vi "PCSLauncher.get Supers and Start-GOGs.vi"(0 "i ref in":refnum<vi>, 5 "error in (no error)":errorcluster) -> (14 "i ref out":refnum<vi>, 16 "Super Instances":string[](array[string]), 17 "Start-GOG Instances":string[](array[string]), 18 "System Names":string[](array[string]), 19 "error out":errorcluster)   [LabVIEW 2014, in "PCSLauncher.lvlib"]
uses:
  PCSLauncher.lvlib
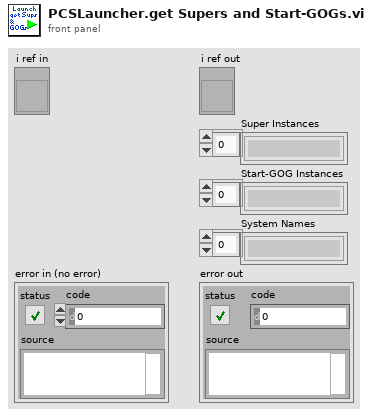
[diagram p1: front panel]
types:
  T1 = typedef "PCSLauncher.lvlib/PCSLauncher.i attribute.ctl" = cluster{"PCS Systems":cluster{"GUI Ref":refnum<vi>, "Super alive?":bool, "Start-GOG alive?":bool}[], "GUI Refs":cluster{"Delete":refnum<vi>, "Launch PCS":refnum<vi>}}
  T2 = cluster{"GUI Ref":refnum<vi>, "Super alive?":bool, "Start-GOG alive?":bool}[]
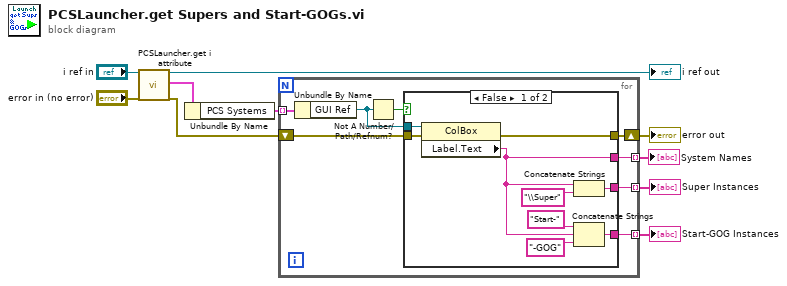
[diagram p0: block diagram]
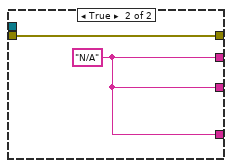
[diagram p2: hidden frame]
diagram:
  n1 = call "PCSLauncher.get i attribute.vi"("i ref in"="i ref in", "error in (no error)"="error in (no error)") -> ("i ref out"=→"i ref out":refnum<vi>, "i attribute"=w5:T1, "error out"=w7:errorcluster)  [unwired: 15 in]
  n2 = Unbundle By Name(w5) -> ("PCS Systems"=w6:T2)
  n3 = for {
    tunnel: w6 -> [w18] mode=indexing
    shift-right: [w14] -> w8
    shift-left: w7 -> [w15]
    tunnel: [w13] -> w9 mode=indexing
    tunnel: [w12] -> w10 mode=indexing
    tunnel: [w11] -> w1 mode=indexing
    n4 = Unbundle By Name(w18) -> ("GUI Ref"=w16:refnum<vi>)
    n5 = Not A Number/Path/Refnum?(number/path/refnum=w16) -> (NaN/Path/Refnum?=w17:bool)
    n6 = case shown="False" w17 {
      tunnel: w16 -> [w27 _]
      tunnel: w15 -> [w26 w29]
      tunnel: [w25 w29] -> w14
      tunnel: [w21 w28] -> w13
      tunnel: [w20 w28] -> w12
      tunnel: [w19 w28] -> w11
      frame False {
        n7 = property class="ColBox"(reference=w27, error in=w26) -> (error out=w25:errorcluster, "Label.Text"=w19:string)  [unwired: 1 out]
        n8 = Concatenate Strings(w19, "\\Super" ("string")) -> (w21:string)
        n9 = Concatenate Strings("Start-" ("string"), w19, "-GOG" ("string")) -> (w20:string)
      }
      frame True {
        w28 = "N/A"
      }
    }
  }
  "Start-GOG Instances" <- w10
  "Super Instances" <- w9
  "error out" <- w8
  "System Names" <- w1
